vi "From Variant.vi"(8 "Error In":errorcluster, 10 "Variant":variant, 11 "TD String A In":refnum<class "1D String.lvclass">) -> (0 "Error Out":errorcluster, 3 "TD String A Out":refnum<class "1D String.lvclass">)   [LabVIEW 2020, in "NI_VIAnCFGDataStructure.lvlib" / "1D String.lvclass"]
doc: "Dynamic dispatch interface for conversion of variant LV data to Tree Data classes."
uses:
  <vilib>/addons/analyzer/VIAnCFGDataStructure/Data Types/String Array/1D String.lvclass
  <vilib>/addons/analyzer/VIAnCFGDataStructure/Data Types/String Array/1D String.lvclass/1D String.ctl
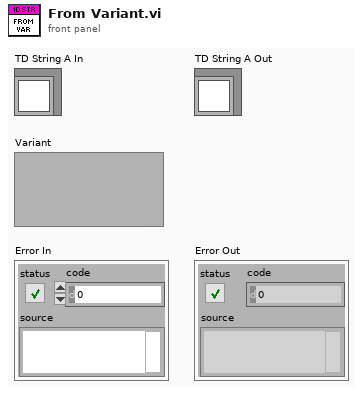
[diagram p1: front panel]
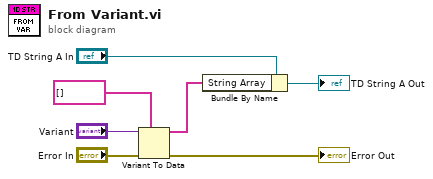
[diagram p0: block diagram]
diagram:
  n1 = Variant To Data(error in="Error In", type=string[] [] ("String Array"), Variant="Variant") -> (data=w2:string[], error out=→"Error Out":errorcluster)
  n2 = Bundle By Name(cluster="TD String A In", "String Array"=w2) -> (→"TD String A Out":refnum<class "1D String.lvclass">)
